vi "find Index and length.vi"(0 "error in (no error)":errorcluster, 11 "number of DRV":i32) -> (2 "length":i32, 3 "index":i32, 8 "error out":errorcluster)   [LabVIEW 2018, in "Application.lvlib"]
uses:
  Application.lvlib
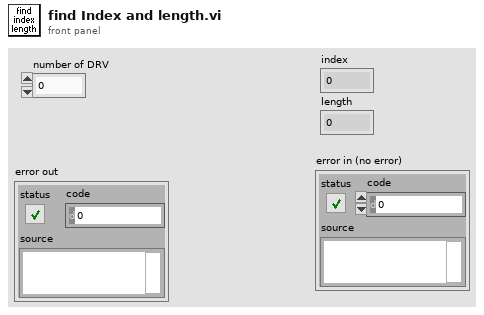
[diagram p1: front panel]
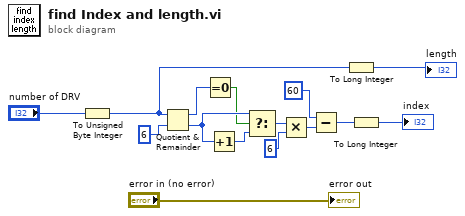
[diagram p0: block diagram]
diagram:
  n1 = To Unsigned Byte Integer(number="number of DRV") -> (unsigned 8bit integer=w1:u8)
  n2 = Quotient & Remainder(x=w1, y=u8 6) -> (x-y*floor(x/y)=w11:u8, floor(x/y)=w10:u8)
  n3 = Equal To 0?(x=w11) -> (x = 0?=w9:bool)
  n4 = Increment(x=w10) -> (x+1=w8:u8)
  n5 = Select(t=w10, s=w9, f=w8) -> (s? t:f=w7:u8)
  n6 = Multiply(x=w7, y=u8 6) -> (x*y=w13:u8)
  n7 = Subtract(x=u8 60, y=w13) -> (x-y=w4:u8)
  n8 = To Long Integer(number=w1) -> (32bit integer=→"length":i32)
  n9 = To Long Integer(number=w4) -> (32bit integer=→"index":i32)
  "error out" <- "error in (no error)"
